vi "Inventory FGV.vi"(7 "error in":errorcluster, 9 "Device Info":T1, 10 "Command":T3(ring)) -> (0 "error out":errorcluster, 2 "Device Info Out":T1, 3 "array of devices":T2)   [LabVIEW 2016]
uses:
  Array Device Info.ctl
  Device Info.ctl
  Globals.vi
  <vilib>/Utility/error.llb/Error Cluster From Error Code.vi
  <vilib>/ErrorRing/Error Ring.xnode
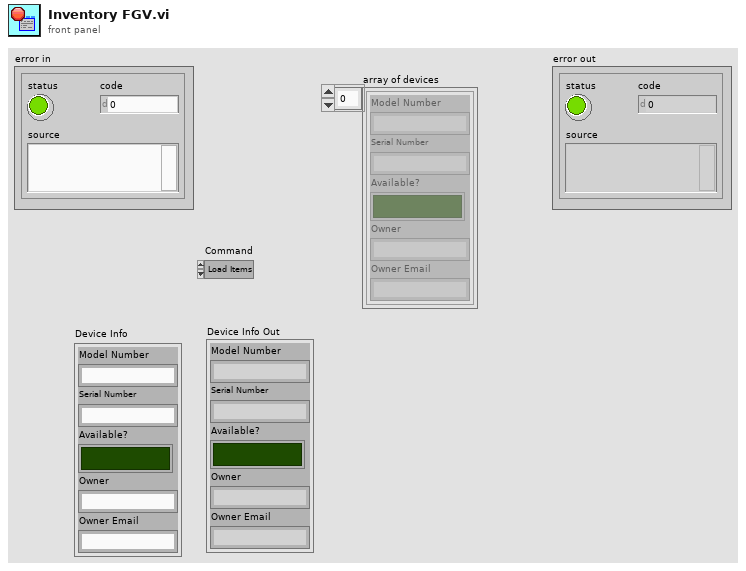
[diagram p1: front panel]
types:
  T1 = typedef "Device Info.ctl" = cluster{"Model Number":string, "Serial Number":string, "Available?":bool, "Owner":string, "Owner Email":string}
  T2 = typedef "Array Device Info.ctl" = T1[]
  T3 = enum16{"Load Items", "Check Status", "Return Items", "Check Out Items", "Add New Item", "Get All Items", "Remove Item"}
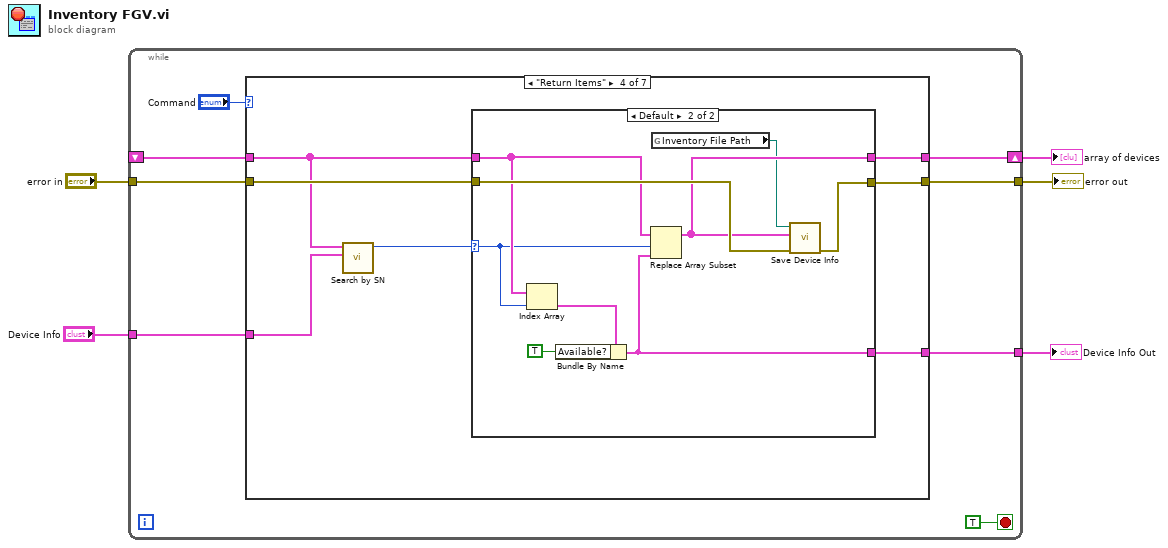
[diagram p0: block diagram]
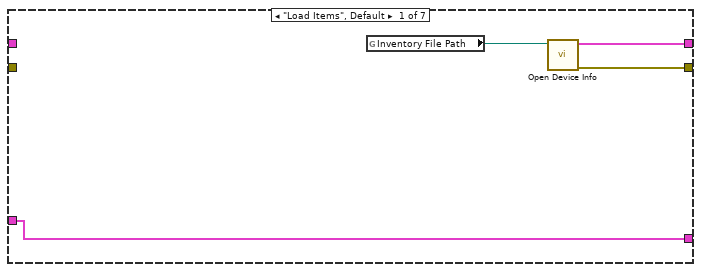
[diagram p2: hidden frame]
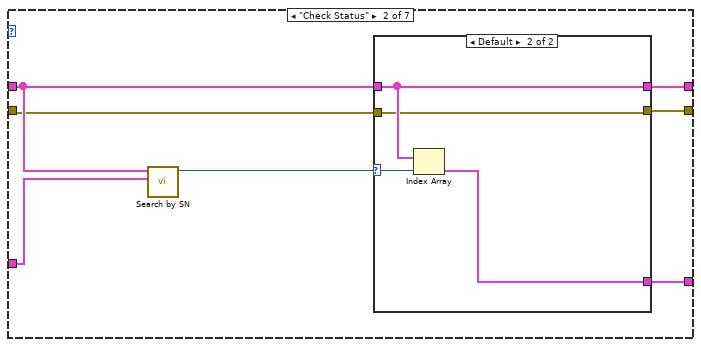
[diagram p3: hidden frame]
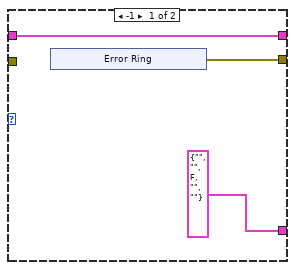
[diagram p4: hidden frame]
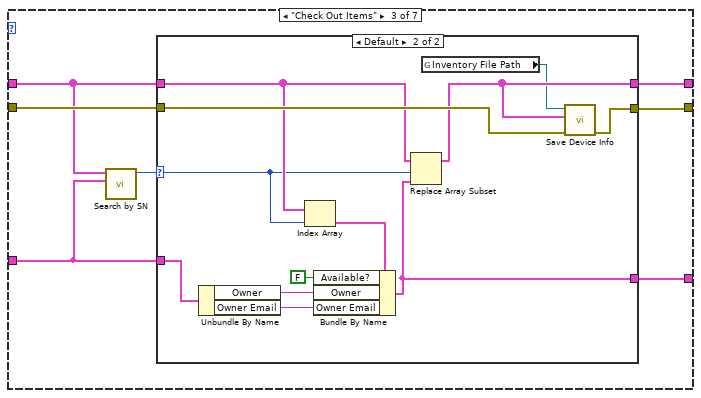
[diagram p5: hidden frame]
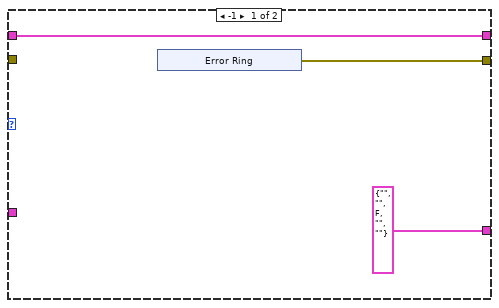
[diagram p6: hidden frame]
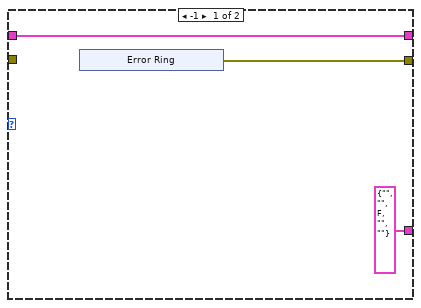
[diagram p7: hidden frame]
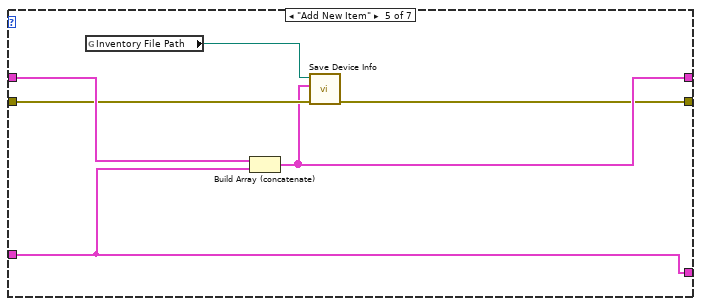
[diagram p8: hidden frame]
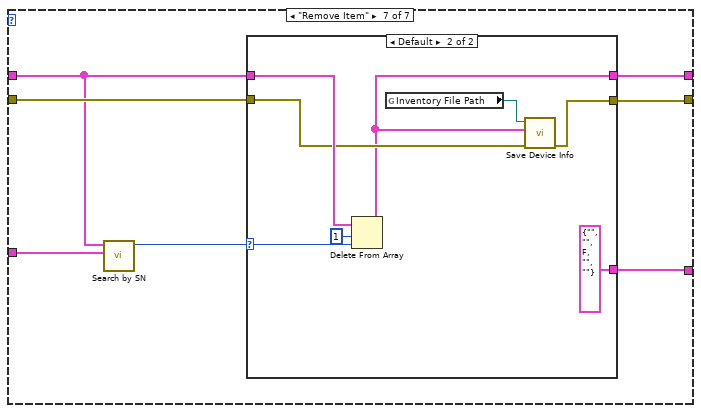
[diagram p10: hidden frame]
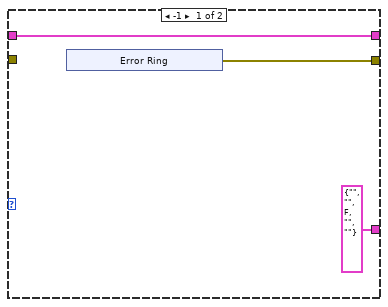
[diagram p11: hidden frame]
diagram:
  n1 = while {
    shift-right: [w11] -> w4
    shift-left: _ -> [w10]
    tunnel: [w9] -> w5
    tunnel: "Device Info" -> [w8]
    tunnel: "error in" -> [w7]
    tunnel: [w6] -> w1
    stop <- TRUE stop-if-true
    n2 = case shown="\"Return Items\"" "Command" {
      tunnel: [w17 w20 w39 w65 w90 w96 w100] -> w11
      tunnel: w10 -> [_ w21 w41 w68 w93 w96 w99]
      tunnel: [w16 w22 w40 w67 w89 w95 w101] -> w9
      tunnel: w8 -> [w14 w24 w37 w66 w88 w94 w97]
      tunnel: w7 -> [_ w19 w42 w69 w91 w95 w102]
      tunnel: [w14 w18 w38 w64 w88 w94 w98] -> w6
      frame "Load Items", Default {
        n3 = global read "Globals.vi" "Inventory File Path"() -> (w15:path)
        n4 = call "Open Device Info.vi"("File Path"=w15) -> ("error out"=w16:errorcluster, "array of devices"=w17:T2)  [unwired: 9 in]
      }
      frame "Check Status" {
        n5 = call "Search by SN.vi"("Device Info"=w24, "array of devices"=w21) -> ("index of element"=w23:i32)  [unwired: 9 in]
        n6 = case shown="Default" w23 {
          selector: w23 -> [_ w35]
          tunnel: [w27 w34] -> w22
          tunnel: w21 -> [w26 w36]
          tunnel: [w26 w36] -> w20
          tunnel: w19 -> [_ w34]
          tunnel: [T1 {"Model Number"="", "Serial Number"="", "Available?"=FALSE, "Owner"="", "Owner Email"=""} ("Device") w33] -> w18
          frame -1 {
            n7 = xnode "Error Ring"() -> ("error out"=w27:errorcluster)
          }
          frame Default {
            n8 = Index Array(array=w36, index=w35) -> (element=w33:T1)
          }
        }
      }
      frame "Check Out Items" {
        n9 = call "Search by SN.vi"("Device Info"=w37, "array of devices"=w41) -> ("index of element"=w43:i32)  [unwired: 9 in]
        n10 = case shown="Default" w43 {
          selector: w43 -> [_ w56]
          tunnel: w42 -> [_ w62]
          tunnel: w41 -> [w45 w57]
          tunnel: [w46 w61] -> w40
          tunnel: [w45 w60] -> w39
          tunnel: [T1 {"Model Number"="", "Serial Number"="", "Available?"=FALSE, "Owner"="", "Owner Email"=""} ("Device") w58] -> w38
          tunnel: w37 -> [_ w54]
          frame -1 {
            n11 = xnode "Error Ring"() -> ("error out"=w46:errorcluster)
          }
          frame Default {
            n12 = Unbundle By Name(w54) -> ("Owner"=w53:string, "Owner Email"=w52:string)
            n13 = Index Array(array=w57, index=w56) -> (element=w55:T1)
            n14 = Bundle By Name(cluster=w55, "Available?"=FALSE ("Loan Status"), "Owner"=w53, "Owner Email"=w52) -> (w58:T1)
            n15 = Replace Array Subset(array=w57, new element=w58, index=w56) -> (w60:T2)
            n16 = global read "Globals.vi" "Inventory File Path"() -> (w59:path)
            n17 = call "Save Device Info.vi"("error in"=w62, "Array of Device Info"=w60, "File Path"=w59) -> ("error out"=w61:errorcluster)  [unwired: 8 in]
          }
        }
      }
      frame "Return Items" {
        n18 = call "Search by SN.vi"("Device Info"=w66, "array of devices"=w68) -> ("index of element"=w70:i32)  [unwired: 9 in]
        n19 = case shown="Default" w70 {
          selector: w70 -> [_ w80]
          tunnel: w69 -> [_ w86]
          tunnel: w68 -> [w72 w81]
          tunnel: [w73 w85] -> w67
          tunnel: [w72 w84] -> w65
          tunnel: [T1 {"Model Number"="", "Serial Number"="", "Available?"=FALSE, "Owner"="", "Owner Email"=""} ("Device") w82] -> w64
          frame -1 {
            n20 = xnode "Error Ring"() -> ("error out"=w73:errorcluster)
          }
          frame Default {
            n21 = Index Array(array=w81, index=w80) -> (element=w79:T1)
            n22 = Bundle By Name(cluster=w79, "Available?"=TRUE ("Loan Status")) -> (w82:T1)
            n23 = Replace Array Subset(array=w81, new element=w82, index=w80) -> (w84:T2)
            n24 = global read "Globals.vi" "Inventory File Path"() -> (w83:path)
            n25 = call "Save Device Info.vi"("error in"=w86, "Array of Device Info"=w84, "File Path"=w83) -> ("error out"=w85:errorcluster)  [unwired: 8 in]
          }
        }
      }
      frame "Add New Item" {
        n26 = global read "Globals.vi" "Inventory File Path"() -> (w92:path)
        n27 = Build Array (concatenate)(w93, w88) -> (w90:T2)
        n28 = call "Save Device Info.vi"("error in"=w91, "Array of Device Info"=w90, "File Path"=w92) -> ("error out"=w89:errorcluster)  [unwired: 8 in]
      }
      frame "Get All Items" {
      }
      frame "Remove Item" {
        n29 = call "Search by SN.vi"("Device Info"=w97, "array of devices"=w99) -> ("index of element"=w103:i32)  [unwired: 9 in]
        n30 = case shown="Default" w103 {
          selector: w103 -> [_ w118]
          tunnel: w102 -> [_ w116]
          tunnel: [w106 w115] -> w101
          tunnel: [w105 w114] -> w100
          tunnel: w99 -> [w105 w119]
          tunnel: [T1 {"Model Number"="", "Serial Number"="", "Available?"=FALSE, "Owner"="", "Owner Email"=""} ("Device Info") T1 {"Model Number"="", "Serial Number"="", "Available?"=FALSE, "Owner"="", "Owner Email"=""} ("Device Info")] -> w98
          frame -1 {
            n31 = xnode "Error Ring"() -> ("error out"=w106:errorcluster)
          }
          frame Default {
            n32 = Delete From Array(array=w119, length=1, index=w118) -> (array with subset deleted=w114:T2)  [unwired: 1 out]
            n33 = global read "Globals.vi" "Inventory File Path"() -> (w113:path)
            n34 = call "Save Device Info.vi"("error in"=w116, "Array of Device Info"=w114, "File Path"=w113) -> ("error out"=w115:errorcluster)  [unwired: 8 in]
          }
        }
      }
    }
  }
  "error out" <- w5
  "array of devices" <- w4
  "Device Info Out" <- w1
